vi "Untitled 1.vi"() -> ()   [LabVIEW 2022 SP3]
uses:
  <vilib>/xnet/xnet.llb/XNET Frame CAN.ctl
  <vilib>/xnet/xnet.llb/XNET Frame Type CAN.ctl
  <vilib>/xnet/xnet.llb/XNET Control Scope.ctl
  <vilib>/xnet/xnet.llb/XNET Create Session (Frame Output Single-point).vi
  <vilib>/xnet/xnet.llb/XNET Create Session (Frame Input Single-point).vi
  <vilib>/xnet/xnet.llb/XNET Write (Frame CAN).vi
  <vilib>/xnet/xnet.llb/XNET Read (Frame CAN).vi
  <resource>/objmgr/xnet.rc
panel:
  out "data":T1[](array[typedef]) {"payload" format="%x"; "timestamp" format="%<%.7X\n%x>T"; "type" items=["CAN Data"=0, "CAN Remote"=1, "CAN Bus Error"=2, "CAN 2.0 Data"=8, "CAN FD Data"=16, "CAN FD+BRS Data"=24, "J1939 Data"=192, "Delay"=224, "Log Trigger"=225, "Start Trigger"=226]; "identifier" format="%x"}
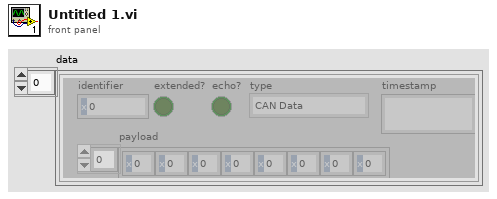
[diagram p1: front panel]
types:
  T1 = typedef "XNET Frame CAN.ctl" = cluster{"timestamp":timestamp, "payload":u8[], "identifier":u32, "type":T2, "extended?":bool, "echo?":bool}
  T2 = typedef "XNET Frame Type CAN.ctl" = u8
  T3 = typedef "XNET Control Scope.ctl" = u32
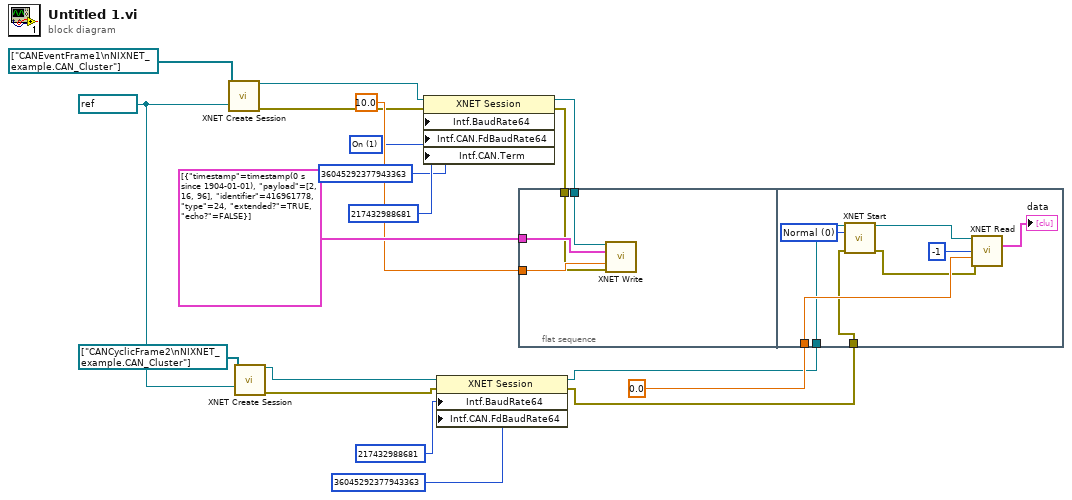
[diagram p0: block diagram]
diagram:
  w7 = u32 1 items=["Off", "On"] ("Interface:CAN:Termination")
  w18 = refnum<k21> "CAN1" ("interface")
  n1 = call-poly <vilib>:"XNET Create Session.vi"("frame list"=refnum<k21>[] ["CANEventFrame1\nNIXNET_example.CAN_Cluster"], "interface"=w18) -> ("session out"=w11:refnum<k21>, "error out"=w10:errorcluster)  [unwired: 12 in]
  n2 = call-poly <vilib>:"XNET Create Session.vi"("frame list"=refnum<k21>[] ["CANCyclicFrame2\nNIXNET_example.CAN_Cluster"], "interface"=w18) -> ("session out"=w6:refnum<k21>, "error out"=w5:errorcluster)  [unwired: 12 in]
  n3 = property class="XNET Session"(reference=w11, error in=w10, "Intf.BaudRate64"=u64 217432988681 ("Interface:64bit Baud Rate"), "Intf.CAN.FdBaudRate64"=u64 36045292377943363 ("Interface:CAN:64bit FD Baud Rate"), "Intf.CAN.Term"=w7) -> (reference out=w9:refnum<k21>, error out=w8:errorcluster)
  n4 = property class="XNET Session"(reference=w6, error in=w5, "Intf.BaudRate64"=u64 217432988681 ("Interface:64bit Baud Rate"), "Intf.CAN.FdBaudRate64"=u64 36045292377943363 ("Interface:CAN:64bit FD Baud Rate")) -> (reference out=w3:refnum<k21>, error out=w4:errorcluster)
  n5 = flat-sequence {
    tunnel: T1[] [{"timestamp"=timestamp(0 s since 1904-01-01), "payload"=[2, 16, 96], "identifier"=416961778, "type"=24, "extended?"=TRUE, "echo?"=FALSE}] ("data") -> [w23]
    tunnel: 10.0 ("timeout (10)") -> [w22]
    tunnel: w9 -> [w21]
    tunnel: w8 -> [w20]
    tunnel: w3 -> [w28]
    tunnel: 0.0 ("timeout (0)") -> [w31]
    tunnel: w4 -> [w27]
    frame #0 {
      n6 = call-poly <vilib>:"XNET Write.vi"("session in"=w21, "data"=w23, "timeout (10)"=w22, "error in (no error)"=w20) -> ()  [unwired: 10 in, 2 out]
    }
    frame #1 {
      w26 = T3 0 items=["Normal", "Session Only", "Interface Only", "Session Only Blocking"] ("scope (normal)")
      n7 = call <vilib>:"XNET Start.vi"("session in"=w28, "scope (normal)"=w26, "error in (no error)"=w27) -> ("session out"=w25:refnum<k21>, "error out"=w24:errorcluster)  [unwired: 11 in]
      n8 = call-poly <vilib>:"XNET Read.vi"("session in"=w25, "number to read (-1)"=-1, "timeout (0)"=w31, "error in (no error)"=w24) -> ("data"=→"data":T1[])  [unwired: 8 in, 3 out]
    }
  }
